vi "UpdateLiquidVolume.vi"(9 "default pulse duration":dbl, 10 "Ring Text.Text":string, 11 "Params":T1={"Mice ID"=[], "ExpType"=[], "Trial Interval"=[], "Pulse Duration"=[158.0, 152.0, 156.0, 167.0, 172.0], "microL_per_pulse"=[6.0, 6.0, 6.0, 6.0, 6.0], "Response Interval"=[1000.0, 1000.0, 1000.0, 1000.0, 1000.0], "Bad Delay"=[], "Response Period"=[], "liquid_type"="water", "Stimuli"=[], "Rewarded Stimuli"=[], "AirDur"=[]} {"AirDur" format="%#_13g"}) -> (2 "Change":bool, 3 "Params 2":T1={"Mice ID"=[], "ExpType"=[], "Trial Interval"=[], "Pulse Duration"=[158.0, 152.0, 156.0, 167.0, 172.0], "microL_per_pulse"=[6.0, 6.0, 6.0, 6.0, 6.0], "Response Interval"=[1000.0, 1000.0, 1000.0, 1000.0, 1000.0], "Bad Delay"=[], "Response Period"=[], "liquid_type"="water", "Stimuli"=[], "Rewarded Stimuli"=[], "AirDur"=[]} {"AirDur" format="%#_13g"})   [LabVIEW 2014]
uses:
  ParamsArray.ctl
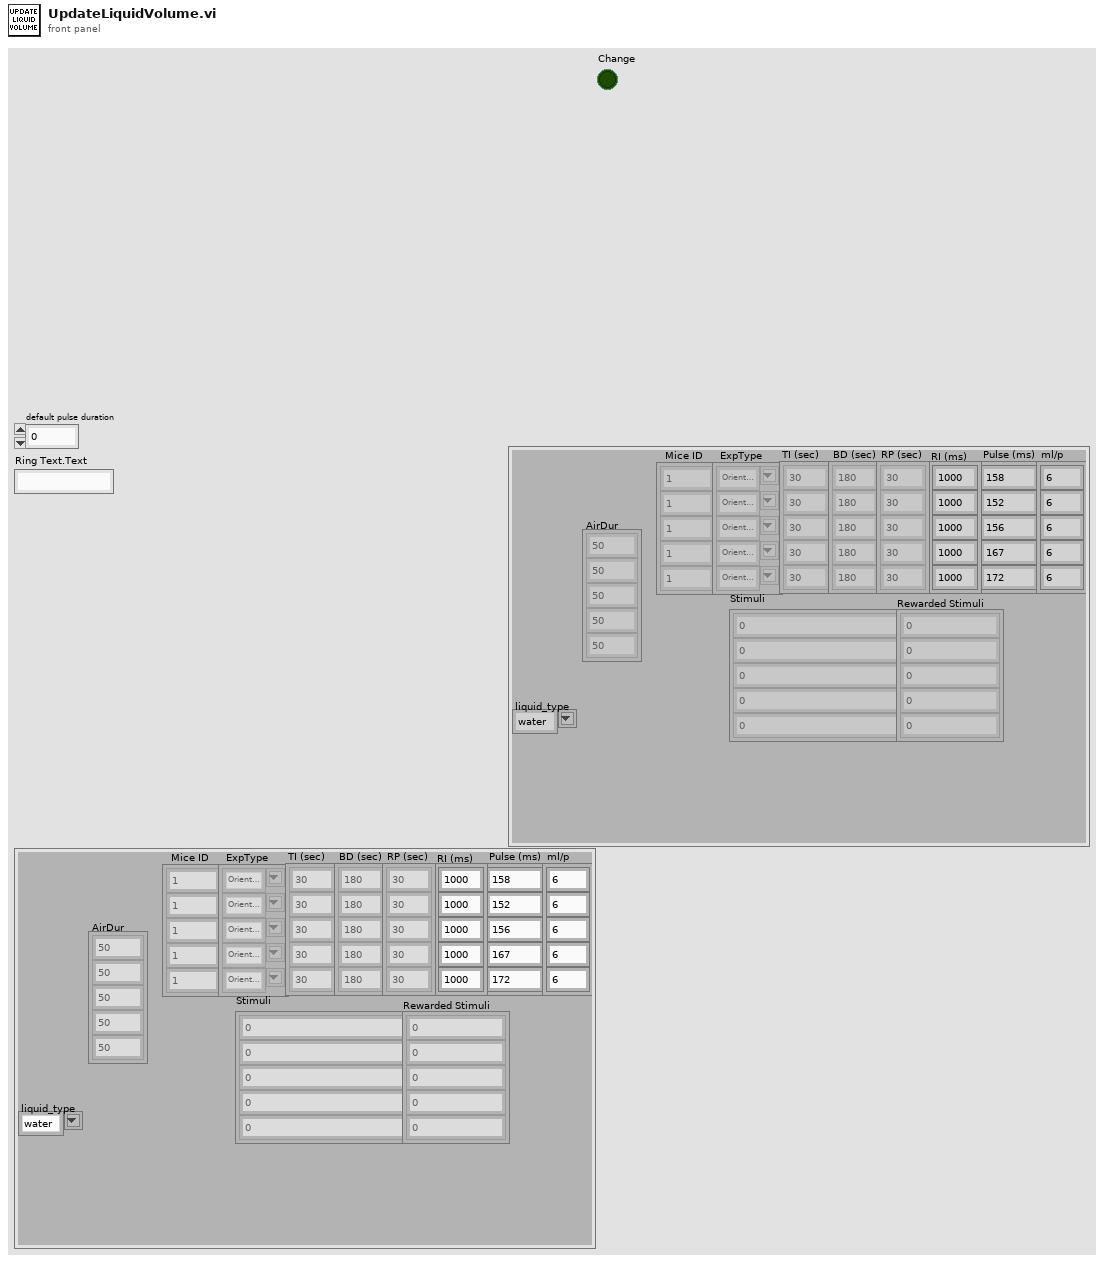
[diagram p1: front panel]
types:
  T1 = typedef "ParamsArray.ctl" = cluster{"Mice ID":dbl[], "ExpType":string[], "Trial Interval":dbl[], "Pulse Duration":dbl[], "microL_per_pulse":dbl[], "Response Interval":dbl[], "Bad Delay":dbl[], "Response Period":dbl[], "liquid_type":string, "Stimuli":string[], "Rewarded Stimuli":string[], "AirDur":dbl[]}
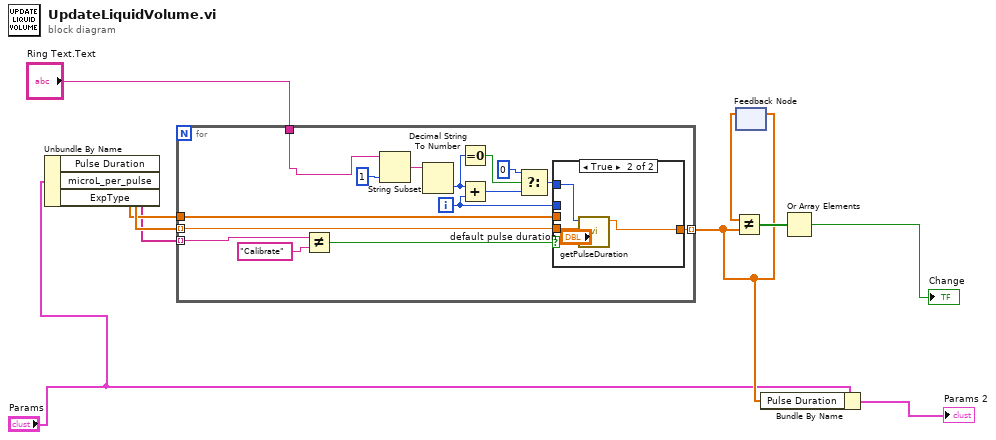
[diagram p0: block diagram]
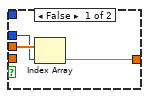
[diagram p2: hidden frame]
diagram:
  n1 = Unbundle By Name("Params") -> ("Pulse Duration"=w9:dbl[], "microL_per_pulse"=w10:dbl[], "ExpType"=w8:string[])
  n2 = for {
    tunnel: w10 -> [w23] mode=indexing
    tunnel: [w21] -> w4 mode=indexing
    tunnel: w9 -> [w13]
    tunnel: w8 -> [w20] mode=indexing
    tunnel: "Ring Text.Text" -> [w11]
    i -> [w12]
    n3 = Not Equal?(x=w20, y="Calibrate") -> (x != y?=w19:bool)
    n4 = String Subset(string=w11, length (rest)=1 ("length (rest)")) -> (substring=w25:string)  [unwired: 1 in]
    n5 = Decimal String To Number(string=w25) -> (number=w16:i32)  [unwired: 2 in, 1 out]
    n6 = Equal To 0?(x=w16) -> (x = 0?=w15:bool)
    n7 = Add(x=w16, y=w12) -> (x+y=w18:i32)
    n8 = Select(t=0, s=w15, f=w18) -> (s? t:f=w17:i32)
    n9 = case shown="True" w19 {
      tunnel: w17 -> [_ w32]
      tunnel: w23 -> [_ w31]
      tunnel: [w26 w30] -> w21
      tunnel: w13 -> [w28 _]
      tunnel: w12 -> [w27 _]
      frame False {
        n10 = Index Array(array=w28, index=w27) -> (element=w26:dbl)
      }
      frame True {
        n11 = call "getPulseDuration.vi"("default pulse duration"="default pulse duration", "target microL/pulse"=w31, "Probe #"=w32) -> ("Pulse Duration"=w30:dbl)  [unwired: 8 in]
      }
    }
  }
  n12 = feedback #1() -> (w7:dbl[])  [unwired: 1 in]
  n13 = Not Equal?(x=w7, y=w4) -> (x != y?=w6:bool[])
  n14 = feedback-in #1(w4) -> ()
  n15 = Bundle By Name(cluster="Params", "Pulse Duration"=w4) -> (→"Params 2":T1)
  n16 = Or Array Elements(Boolean array=w6) -> (logical OR=→"Change":bool)
